vi "Populate HEWH Commands.vi"() -> (2 "GEA2 Command Table":string[][](array[string]), 3 "GEA2 Command Cluster":T2(array[cluster]) {"CMD Array" format="%x"; "Destination" format="%x"})   [LabVIEW 2018]
uses:
  Type Definitions/GEA2 Commands.ctl
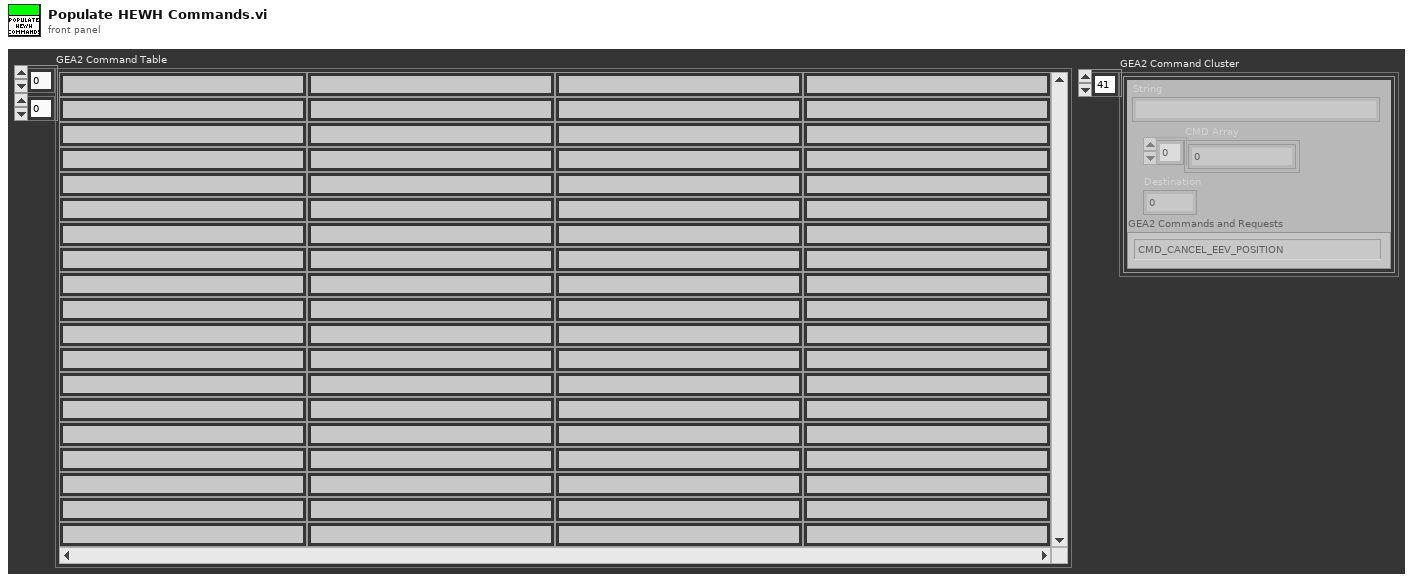
[diagram p1: front panel]
types:
  T1 = typedef "GEA2 Commands.ctl" = enum16{"CMD_CANCEL_EEV_POSITION", "CMD_CLEAR_ENERGY_USAGE_CTRS", "CMD_CLEAR_FAULT_COUNTS", "CMD_CLEAR_OVERRIDE_STATUS", "CMD_COMP_OFF", "CMD_COMP_ON", "CMD_DSM_OVERRIDES", "CMD_EEV_POSITION", "CMD_ENTER_EXIT_FCT_MODE", "CMD_ENTER_FACT_MODE", "CMD_HP_RUN_6MIN", "CMD_INITIATE_REMOTE_DSM_OVERRIDE", "CMD_LE_2_SECONDS", "CMD_REFRESH_SERVICE_TIMEOUTS", "CMD_RESET", "CMD_RESET_FILTER_TIMES", "CMD_RESTORE_EEPROM_DEFAULTS", "CMD_RQST_LED_STATUS", "CMD_SET_AMBIENT_THRESH_1", "CMD_SET_AMBIENT_THRESH_2", "CMD_SET_AMBIENT_THRESH_3", "CMD_SET_CURRENTS", "CMD_SET_EEV_DRIVE_LINES", "CMD_SET_EEV_STOP_POSITION", "CMD_SET_LEDS", "CMD_SET_MODEL_NUMBER", "CMD_SET_PID_I_DENOM_OVER_THR", "CMD_SET_PID_I_DENOM_UNDER_THR", "CMD_SET_PID_LOW_SH_TARGET", "CMD_SET_PID_MID_SH_TARGET", "CMD_SET_PID_P_DENOMINATOR", "CMD_SET_SERIAL_NUMBER", "CMD_SET_START_POS_OVER_THR", "CMD_SET_START_POS_UNDER_THR", "CMD_TOGGLE_FAN", "CMD_TOGGLE_LE_SERV", "CMD_TOGGLE_SERVICE_MODE", "CMD_TOGGLE_UE_SERV", "CMD_TURN_ON_OFF_DLB", "CMD_UE_2_SECONDS", "CMD_UPDATE_DSM_LEVEL", "CMD_UPDATE_MODE", "CMD_WRITE_SETPOINTS", "REQ_READ_KEY_STATUS", "REQ_SYSTEM_MODE", "RQST_CURRENT_PID_SH_TARGET", "RQST_DATA_FROM_DATA_FLASH", "RQST_DATA_FROM_MEMORY", "RQST_DSM_OVERRIDE_STATUS", "RQST_HEM_KWH_DATA", "RQST_HYPERTERM_OUTPUT_DATA", "RQST_IDLB_RESISTANCE", "RQST_MODEL_NUMBER", "RQST_MODEL_SELECT_AD_VALUE", "RQST_OTHER_FAULT_COUNTS", "RQST_OVERRIDE_STATUS", "RQST_PID_PARAMETERS", "RQST_READ_PERSONALITY", "RQST_SERIAL_NUMBER", "RQST_SERVICE_ERROR_CODES", "RQST_Software_Version", "RQST_SS_FAULT_COUNTS", "RQST_STATUS_QUERY", "RQST_STD_ELEC_RANGE", "RQST_SUPPORTED_MODES", "RQST_T2_RESISTANCE", "RQST_T3B_RESISTANCE", "RQST_T4_RESISTANCE", "RQST_T5_RESISTANCE", "RQST_TEMP_RANGE", "RQST_VACATION_RANGE", "RQST_WATER_CAPACITY"}
  T2 = cluster{"String":string, "CMD Array":u8[], "Destination":u8, "GEA2 Commands and Requests":T1}[]
  T3 = cluster{"String":string, "CMD Array":u8[], "Destination":u8, "GEA2 Commands and Requests":T1}
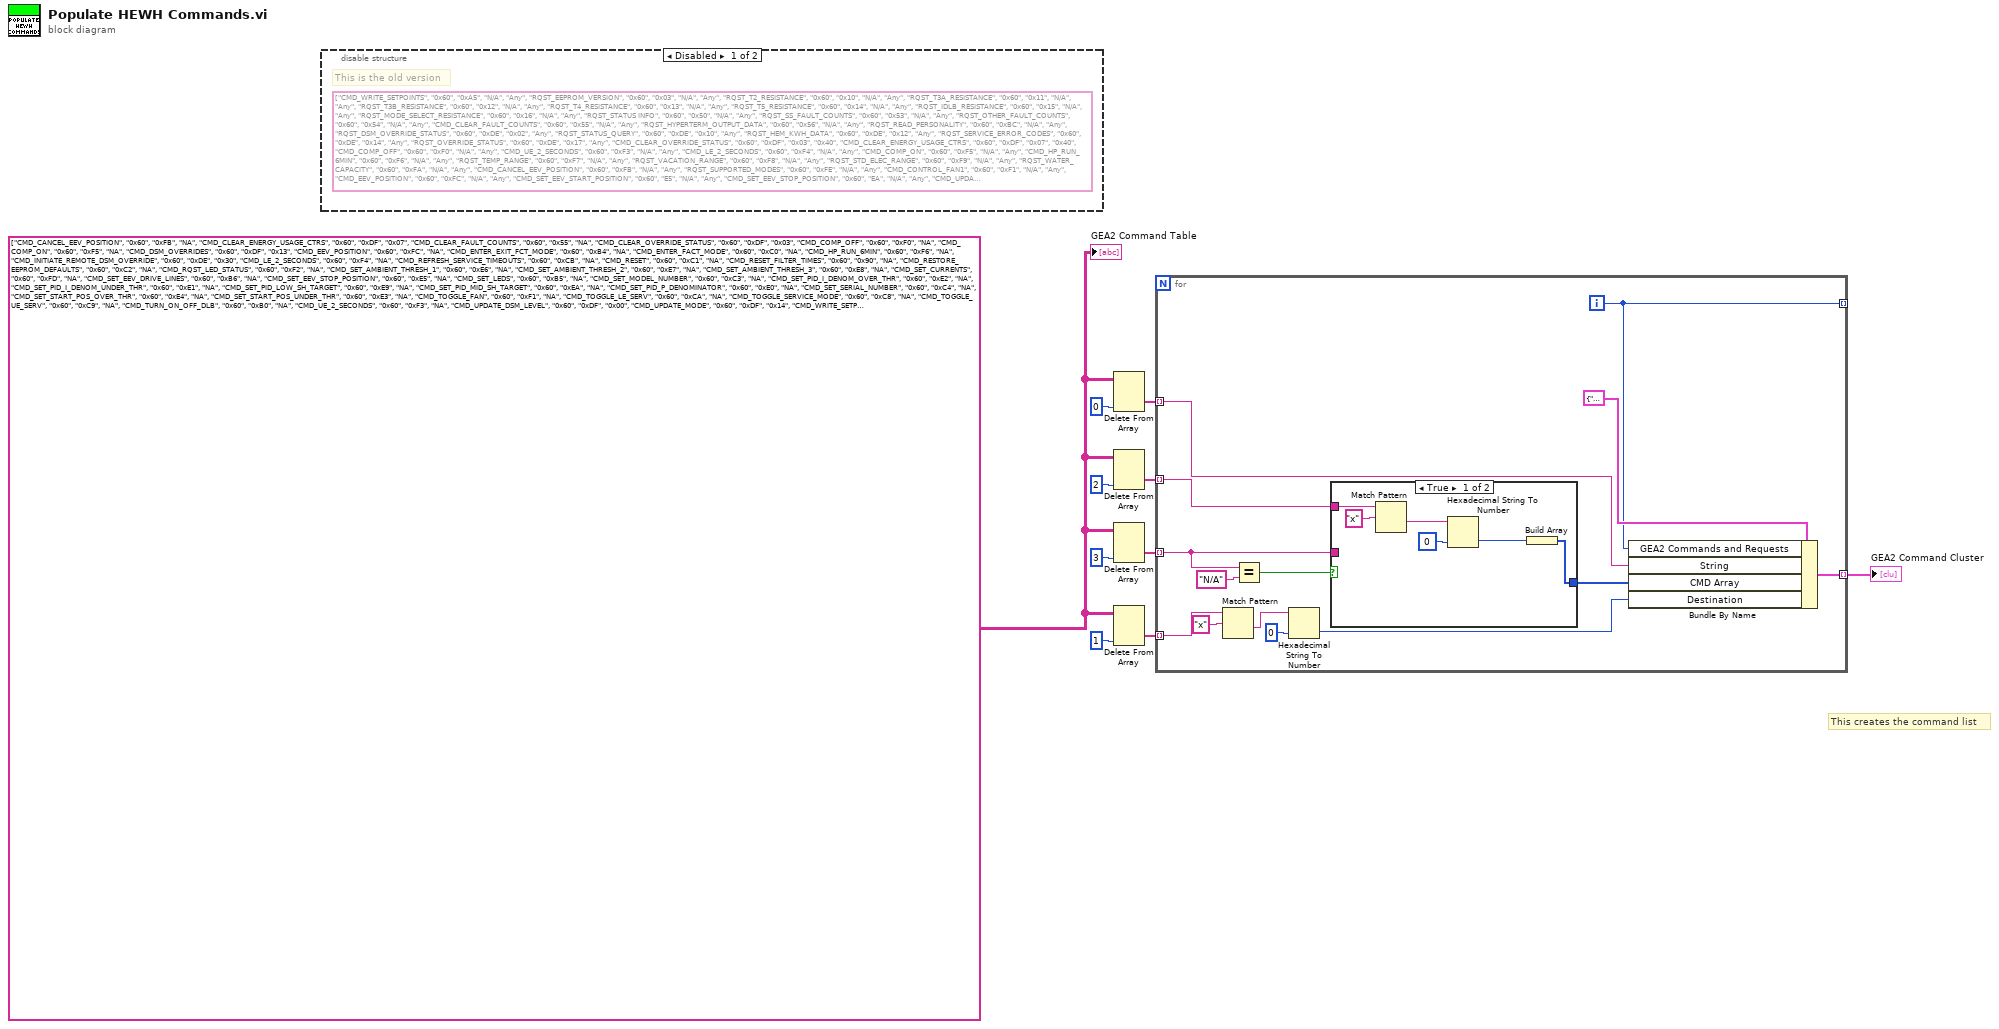
[diagram p0: block diagram]
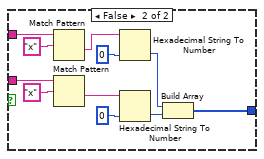
[diagram p3: hidden frame]
diagram:
  w6 = string[][] [["CMD_CANCEL_EEV_POSITION", "0x60", "0xFB", "NA"], ["CMD_CLEAR_ENERGY_USAGE_CTRS", "0x60", "0xDF", "0x07"], ["CMD_CLEAR_FAULT_COUNTS", "0x60", "0x55", "NA"], ["CMD_CLEAR_OVERRIDE_STATUS", "0x60", "0xDF", "0x03"], ["CMD_COMP_OFF", "0x60", "0xF0", "NA"], ["CMD_COMP_ON", "0x60", "0xF5", "NA"], ["CMD_DSM_OVERRIDES", "0x60", "0xDF", "0x13"], ["CMD_EEV_POSITION", "0x60", "0xFC", "NA"], ["CMD_ENTER_EXIT_FCT_MODE", "0x60", "0xB4", "NA"], ["CMD_ENTER_FACT_MODE", "0x60", "0xC0", "NA"], ["CMD_HP_RUN_6MIN", "0x60", "0xF6", "NA"], ["CMD_INITIATE_REMOTE_DSM_OVERRIDE", "0x60", "0xDE", "0x30"], ["CMD_LE_2_SECONDS", "0x60", "0xF4", "NA"], ["CMD_REFRESH_SERVICE_TIMEOUTS", "0x60", "0xCB", "NA"], ["CMD_RESET", "0x60", "0xC1", "NA"], ["CMD_RESET_FILTER_TIMES", "0x60", "0x90", "NA"], ["CMD_RESTORE_EEPROM_DEFAULTS", "0x60", "0xC2", "NA"], ["CMD_RQST_LED_STATUS", "0x60", "0xF2", "NA"], ["CMD_SET_AMBIENT_THRESH_1", "0x60", "0xE6", "NA"], ["CMD_SET_AMBIENT_THRESH_2", "0x60", "0xE7", "NA"], ["CMD_SET_AMBIENT_THRESH_3", "0x60", "0xE8", "NA"], ["CMD_SET_CURRENTS", "0x60", "0xFD", "NA"], ["CMD_SET_EEV_DRIVE_LINES", "0x60", "0xB6", "NA"], ["CMD_SET_EEV_STOP_POSITION", "0x60", "0xE5", "NA"], ["CMD_SET_LEDS", "0x60", "0xB5", "NA"], ["CMD_SET_MODEL_NUMBER", "0x60", "0xC3", "NA"], ["CMD_SET_PID_I_DENOM_OVER_THR", "0x60", "0xE2", "NA"], ["CMD_SET_PID_I_DENOM_UNDER_THR", "0x60", "0xE1", "NA"], ["CMD_SET_PID_LOW_SH_TARGET", "0x60", "0xE9", "NA"], ["CMD_SET_PID_MID_SH_TARGET", "0x60", "0xEA", "NA"], ["CMD_SET_PID_P_DENOMINATOR", "0x60", "0xE0", "NA"], ["CMD_SET_SERIAL_NUMBER", "0x60", "0xC4", "NA"], ["CMD_SET_START_POS_OVER_THR", "0x60", "0xE4", "NA"], ["CMD_SET_START_POS_UNDER_THR", "0x60", "0xE3", "NA"], ["CMD_TOGGLE_FAN", "0x60", "0xF1", "NA"], ["CMD_TOGGLE_LE_SERV", "0x60", "0xCA", "NA"], ["CMD_TOGGLE_SERVICE_MODE", "0x60", "0xC8", "NA"], ["CMD_TOGGLE_UE_SERV", "0x60", "0xC9", "NA"], ["CMD_TURN_ON_OFF_DLB", "0x60", "0xB0", "NA"], ["CMD_UE_2_SECONDS", "0x60", "0xF3", "NA"], ["CMD_UPDATE_DSM_LEVEL", "0x60", "0xDF", "0x00"], ["CMD_UPDATE_MODE", "0x60", "0xDF", "0x14"], ["CMD_WRITE_SETPOINTS", "0x60", "0xA5", "NA"], ["REQ_READ_KEY_STATUS", "0x60", "0xB7", "NA"], ["REQ_SYSTEM_MODE", "0x60", "0xCE", "NA"], ["RQST_CURRENT_PID_SH_TARGET", "0x60", "0xEC", "NA"], ["RQST_DATA_FROM_DATA_FLASH", "0x60", "0x4F", "NA"], ["RQST_DATA_FROM_MEMORY", "0x60", "0x4E", "NA"], ["RQST_DSM_OVERRIDE_STATUS", "0x60", "0xDE", "0x02"], ["RQST_HEM_KWH_DATA", "0x60", "0xDE", "0x12"], ["RQST_HYPERTERM_OUTPUT_DATA", "0x60", "0x56", "NA"], ["RQST_IDLB_RESISTANCE", "0x60", "0x15", "NA"], ["RQST_MODEL_NUMBER", "0x60", "0xC5", "NA"], ["RQST_MODEL_SELECT_AD_VALUE", "0x60", "0x16", "NA"], ["RQST_OTHER_FAULT_COUNTS", "0x60", "0x54", "NA"], ["RQST_OVERRIDE_STATUS", "0x60", "0xDE", "0x17"], ["RQST_PID_PARAMETERS", "0x60", "0xEF", "NA"], ["RQST_READ_PERSONALITY", "0x60", "0xBC", "NA"], ["RQST_SERIAL_NUMBER", "0x60", "0xC6", "NA"], ["RQST_SERVICE_ERROR_CODES", "0x60", "0xDE", "0x14"], ["RQST_Software_Version", "0x60", "0x01", "NA"], ["RQST_SS_FAULT_COUNTS", "0x60", "0x53", "NA"], ["RQST_STATUS_QUERY", "0x60", "0xDE", "0x10"], ["RQST_STD_ELEC_RANGE", "0x60", "0xF9", "NA"], ["RQST_SUPPORTED_MODES", "0x60", "0xFE", "NA"], ["RQST_T2_RESISTANCE", "0x60", "0x10", "NA"], ["RQST_T3B_RESISTANCE", "0x60", "0x12", "NA"], ["RQST_T4_RESISTANCE", "0x60", "0x13", "NA"], ["RQST_T5_RESISTANCE", "0x60", "0x14", "NA"], ["RQST_TEMP_RANGE", "0x60", "0xF7", "NA"], ["RQST_VACATION_RANGE", "0x60", "0xF8", "NA"], ["RQST_WATER_CAPACITY", "0x60", "0xFA", "NA"]] ("all rows 2")
  # "This creates the command list"
  n1 = disable-structure shown="Disabled" {
    frame Disabled {
      (unwired) string[][] [["CMD_WRITE_SETPOINTS", "0x60", "0xA5", "N/A", "Any"], ["RQST_EEPROM_VERSION", "0x60", "0x03", "N/A", "Any"], ["RQST_T2_RESISTANCE", "0x60", "0x10", "N/A", "Any"], ["RQST_T3A_RESISTANCE", "0x60", "0x11", "N/A", "Any"], ["RQST_T3B_RESISTANCE", "0x60", "0x12", "N/A", "Any"], ["RQST_T4_RESISTANCE", "0x60", "0x13", "N/A", "Any"], ["RQST_T5_RESISTANCE", "0x60", "0x14", "N/A", "Any"], ["RQST_IDLB_RESISTANCE", "0x60", "0x15", "N/A", "Any"], ["RQST_MODE_SELECT_RESISTANCE", "0x60", "0x16", "N/A", "Any"], ["RQST_STATUS INFO", "0x60", "0x50", "N/A", "Any"], ["RQST_SS_FAULT_COUNTS", "0x60", "0x53", "N/A", "Any"], ["RQST_OTHER_FAULT_COUNTS", "0x60", "0x54", "N/A", "Any"], ["CMD_CLEAR_FAULT_COUNTS", "0x60", "0x55", "N/A", "Any"], ["RQST_HYPERTERM_OUTPUT_DATA", "0x60", "0x56", "N/A", "Any"], ["RQST_READ_PERSONALITY", "0x60", "0xBC", "N/A", "Any"], ["RQST_DSM_OVERRIDE_STATUS", "0x60", "0xDE", "0x02", "Any"], ["RQST_STATUS_QUERY", "0x60", "0xDE", "0x10", "Any"], ["RQST_HEM_KWH_DATA", "0x60", "0xDE", "0x12", "Any"], ["RQST_SERVICE_ERROR_CODES", "0x60", "0xDE", "0x14", "Any"], ["RQST_OVERRIDE_STATUS", "0x60", "0xDE", "0x17", "Any"], ["CMD_CLEAR_OVERRIDE_STATUS", "0x60", "0xDF", "0x03", "0x40"], ["CMD_CLEAR_ENERGY_USAGE_CTRS", "0x60", "0xDF", "0x07", "0x40"], ["CMD_COMP_OFF", "0x60", "0xF0", "N/A", "Any"], ["CMD_UE_2_SECONDS", "0x60", "0xF3", "N/A", "Any"], ["CMD_LE_2_SECONDS", "0x60", "0xF4", "N/A", "Any"], ["CMD_COMP_ON", "0x60", "0xF5", "N/A", "Any"], ["CMD_HP_RUN_6MIN", "0x60", "0xF6", "N/A", "Any"], ["RQST_TEMP_RANGE", "0x60", "0xF7", "N/A", "Any"], ["RQST_VACATION_RANGE", "0x60", "0xF8", "N/A", "Any"], ["RQST_STD_ELEC_RANGE", "0x60", "0xF9", "N/A", "Any"], ["RQST_WATER_CAPACITY", "0x60", "0xFA", "N/A", "Any"], ["CMD_CANCEL_EEV_POSITION", "0x60", "0xFB", "N/A", "Any"], ["RQST_SUPPORTED_MODES", "0x60", "0xFE", "N/A", "Any"], ["CMD_CONTROL_FAN1", "0x60", "0xF1", "N/A", "Any"], ["CMD_EEV_POSITION", "0x60", "0xFC", "N/A", "Any"], ["CMD_SET_EEV_START_POSITION", "0x60", "E5", "N/A", "Any"], ["CMD_SET_EEV_STOP_POSITION", "0x60", "EA", "N/A", "Any"], ["CMD_UPDATE_DSM_LEVEL", "0x60", "0xDF", "0x00", "0x40"], ["CMD_SET_PID_I_DENOMINATOR", "0x60", "E3", "N/A", "Any"], ["CMD_SET_PID_I_NUMERATOR", "0x60", "E2", "N/A", "Any"], ["RQST_DATA_FROM_MEMORY", "0x60", "0x4E", "N/A", "Any"], ["CMD_OVERRIDE_STATUS_CHANGED", "0x40", "0xDF", "0x02", "0x60"], ["CMD_SET_PID_P_DENOMINATOR", "0x60", "E1", "N/A", "Any"], ["CMD_SET_PID_P_NUMERATOR", "0x60", "E0", "N/A", "Any"], ["CMD_SET_PID_RUN_SH_TARGET", "0x60", "E9", "N/A", "Any"], ["CMD_SET_PID_START_DWELL_TIME", "0x60", "E6", "N/A", "Any"], ["CMD_SET_PID_TRANSITION_TIME", "0x60", "E8", "N/A", "Any"], ["CMD_SET_PID_TRANS_SH_TARGET", "0x60", "E7", "N/A", "Any"], ["CMD_SET_PID_UPDATE_RATE", "0x60", "E4", "N/A", "Any"], ["RQST_DATA_FROM_DATA_FLASH", "0x60", "0x4F", "N/A", "Any"], ["CMD_DSM_OVERRIDES", "0x60", "0xDF", "0x13", "Any"], ["CMD_UPDATE_MODE", "0x60", "0xDF", "0x14", "Any"], ["CMD_UPDATE_SPECIAL_OPERATION", "0x60", "0xDF", "0x15", "Any"], ["CMD_SET_CURRENTS", "0x60", "0xFD", "N/A", "Any"], ["CMD_RESET_FILTER_TIMES", "0x60", "0x90", "N/A", "Any"], ["CMD_TURN_ON_DLB", "0x60", "B0", "N/A", "Any"], ["RQST_PID_PARAMETERS", "0x60", "EF", "N/A", "Any"], ["CMD_CHECK_CRC", "0x60", "0xA6", "N/A", "Any"], ["CMD_ENTER_FACT_MODE", "0x60", "0xC0", "N/A", "Any"], ["CMD_RESET", "0x60", "0xC1", "N/A", "Any"], ["CMD_RESTORE_EEPROM_DEFAULTS", "0x60", "0xC2", "N/A", "Any"], ["RQST_SOFTWARE_VERSION", "0x60", "0x01", "N/A", "0x01"]] ("Data Array 2")
      # "This is the old version"
    }
    frame Enabled {
    }
  }
  n2 = Delete From Array(array=w6, index (col)=0 ("disabled index (col)")) -> (deleted portion=w4:string[])  [unwired: 2 in, 1 out]
  n3 = Delete From Array(array=w6, index (col)=2 ("disabled index (col)")) -> (deleted portion=w3:string[])  [unwired: 2 in, 1 out]
  n4 = Delete From Array(array=w6, index (col)=3 ("disabled index (col)")) -> (deleted portion=w2:string[])  [unwired: 2 in, 1 out]
  n5 = Delete From Array(array=w6, index (col)=1 ("disabled index (col)")) -> (deleted portion=w1:string[])  [unwired: 2 in, 1 out]
  n6 = for {
    tunnel: w4 -> [w12] mode=indexing
    tunnel: w3 -> [w23] mode=indexing
    tunnel: w2 -> [w19] mode=indexing
    tunnel: w1 -> [w15] mode=indexing
    tunnel: [w13] -> w5 mode=indexing
    tunnel: [w11] -> _ mode=indexing
    i -> [w11]
    n7 = Match Pattern(string=w15, regular expression="x") -> (after substring=w17:string)  [unwired: 1 in, 3 out]
    n8 = Equal?(x=w19, y="N/A") -> (x = y?=w20:bool)
    n9 = Hexadecimal String To Number(string=w17, default (0uL)=u8 0 ("default (0 U32)")) -> (number=w14:u8)  [unwired: 1 in, 1 out]
    n10 = case shown="True" w20 {
      tunnel: w23 -> [w30 w41]
      tunnel: [w25 w37] -> w22
      tunnel: w19 -> [_ w35]
      frame True {
        n11 = Match Pattern(string=w30, regular expression="x") -> (after substring=w28:string)  [unwired: 1 in, 3 out]
        n12 = Hexadecimal String To Number(string=w28, default (0uL)=u8 0 ("default (0 U32)")) -> (number=w26:u8)  [unwired: 1 in, 1 out]
        n13 = Build Array(w26) -> (w25:u8[])
      }
      frame False {
        n14 = Match Pattern(string=w41, regular expression="x") -> (after substring=w39:string)  [unwired: 1 in, 3 out]
        n15 = Match Pattern(string=w35, regular expression="x") -> (after substring=w32:string)  [unwired: 1 in, 3 out]
        n16 = Hexadecimal String To Number(string=w39, default (0uL)=u8 0 ("default (0 U32)")) -> (number=w38:u8)  [unwired: 1 in, 1 out]
        n17 = Hexadecimal String To Number(string=w32, default (0uL)=u8 0 ("default (0 U32)")) -> (number=w31:u8)  [unwired: 1 in, 1 out]
        n18 = Build Array(w38, w31) -> (w37:u8[])
      }
    }
    n19 = Bundle By Name(cluster=T3 {"String"="100 Hz", "CMD Array"=[], "Destination"=0, "GEA2 Commands and Requests"=enum."CMD_UPDATE_MODE"}, "GEA2 Commands and Requests"=w11, "String"=w12, "CMD Array"=w22, "Destination"=w14) -> (w13:T3)
  }
  "GEA2 Command Cluster" <- w5
  "GEA2 Command Table" <- w6
